vi "existDevice.vi"(10 "Device":string, 11 "Item Names":string[](array[string])) -> (2 "index":i32, 3 "exist?":bool)   [LabVIEW 2010]
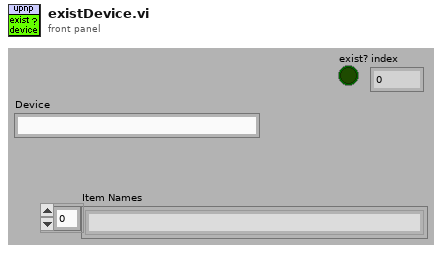
[diagram p1: front panel]
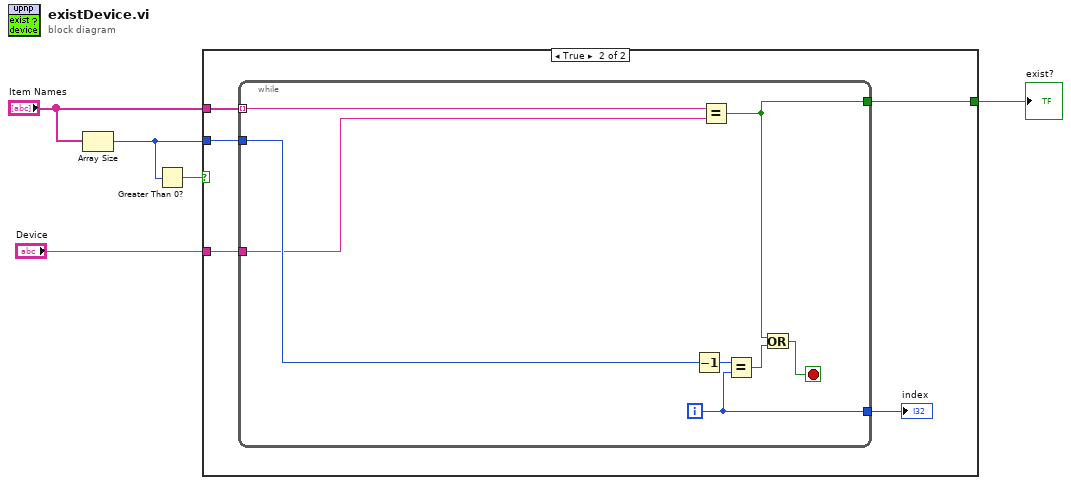
[diagram p0: block diagram]
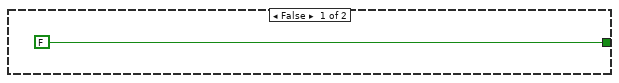
[diagram p2: hidden frame]
diagram:
  n1 = Array Size(array="Item Names") -> (size(s)=w4:i32)
  n2 = Greater Than 0?(x=w4) -> (x > 0?=w2:bool)
  n3 = case shown="True" w2 {
    tunnel: "Item Names" -> [_ w11]
    tunnel: w4 -> [_ w10]
    tunnel: [FALSE w9] -> w3
    tunnel: "Device" -> [_ w8]
    frame False {
    }
    frame True {
      n4 = while {
        tunnel: w11 -> [w12] mode=indexing
        tunnel: [w16] -> w9
        tunnel: w10 -> [w15]
        tunnel: w8 -> [w14]
        tunnel: [w13] -> w7
        i -> [w13]
        stop <- w19 stop-if-true
        n5 = Decrement(x=w15) -> (x-1=w18:i32)
        n6 = Equal?(x=w12, y=w14) -> (x = y?=w16:bool)
        n7 = Equal?(x=w18, y=w13) -> (x = y?=w17:bool)
        n8 = Or(x=w16, y=w17) -> (x .or. y?=w19:bool)
      }
      "index" <- w7
    }
  }
  "exist?" <- w3
